vi "GetCoeffsDomains_v1.vi"(0 "R_H coeffs file":path, 1 "Field index":u16, 2 "Fields":string[](array[string]), 5 "R_H domain file":path, 7 "R_C1 coeffs file":path, 9 "R_C1 domain file":path, 11 "R_C2 coeffs file":path, 12 "R_C2 domain file":path) -> (4 "R_H coeffs":dbl[](array[numeric]), 6 "R_H Log Domain":dbl[](array[numeric]), 8 "R_C1 coeffs":dbl[](array[numeric]), 10 "R_C1 Log Domain":dbl[](array[numeric]), 14 "R_C2 Log Domain":dbl[](array[numeric]), 15 "R_C2 coeffs":dbl[](array[numeric]))   [LabVIEW 2020]
uses:
  <vilib>/Utility/file.llb/Read Delimited Spreadsheet (DBL).vi
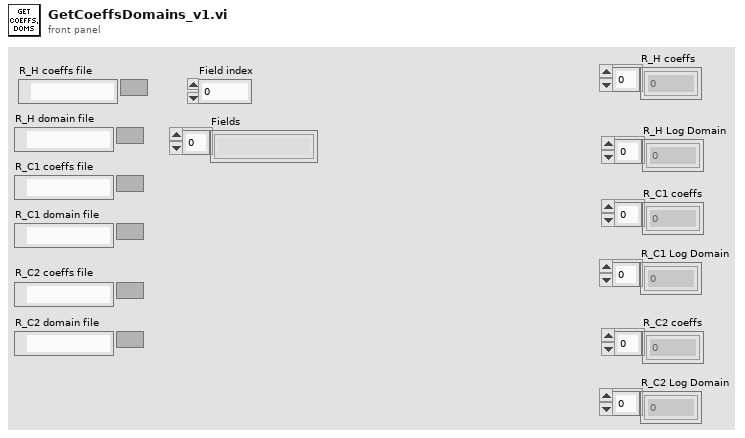
[diagram p1: front panel]
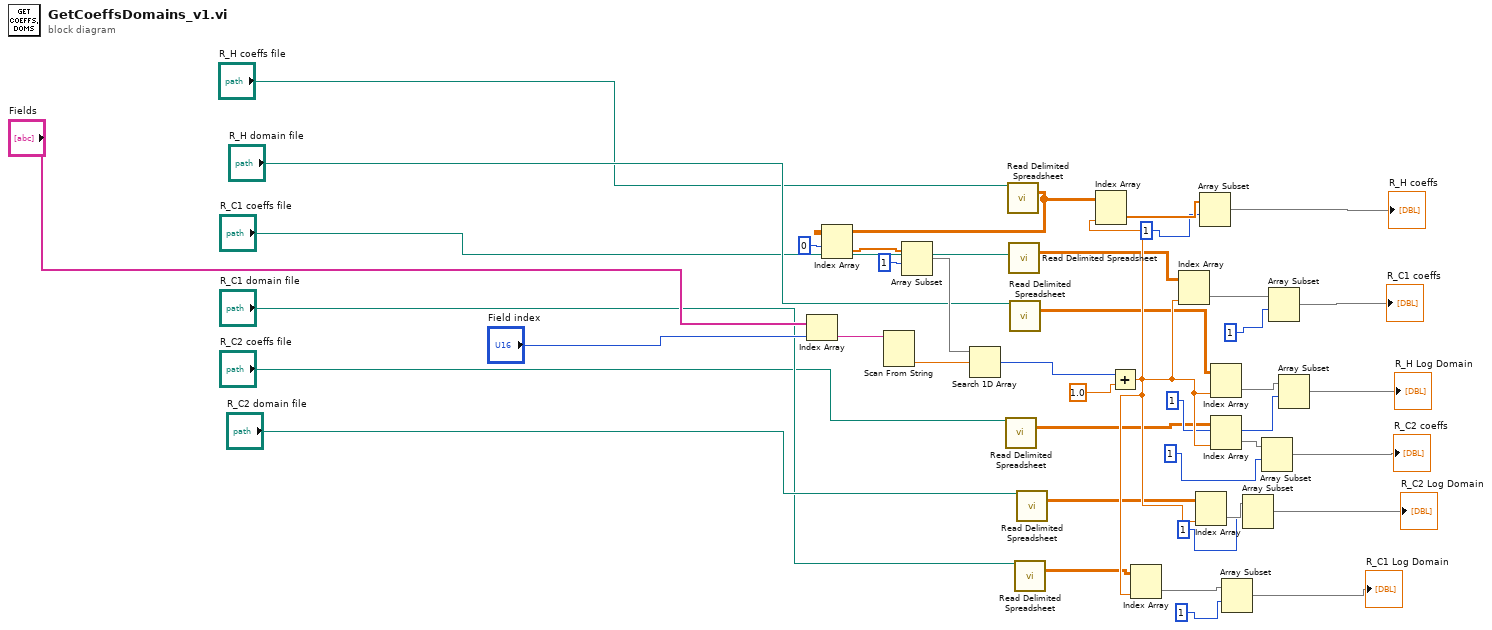
[diagram p0: block diagram]
diagram:
  n1 = Index Array(array="Fields", index="Field index") -> (element=w14:string)
  n2 = Scan From String(input string=w14) -> (output 1=w16:dbl)  [unwired: 4 in, 3 out]
  n3 = call-poly <vilib>:"Read Delimited Spreadsheet.vi"("file path (dialog if empty)"="R_C2 coeffs file") -> ("all rows"=w6:dbl[][])  [unwired: 9 in, 5 out]
  n4 = call-poly <vilib>:"Read Delimited Spreadsheet.vi"("file path (dialog if empty)"="R_H coeffs file") -> ("all rows"=w2:dbl[][])  [unwired: 9 in, 5 out]
  n5 = Index Array(array=w2, index (row)=0) -> (element=w20:dbl[])  [unwired: 1 in]
  n6 = Array Subset(array=w20, index=1) -> (w22:dbl[])  [unwired: 1 in]
  n7 = Search 1D Array(1D array=w22, element=w16) -> (index of element=w24:i32)  [unwired: 1 in]
  n8 = call-poly <vilib>:"Read Delimited Spreadsheet.vi"("file path (dialog if empty)"="R_C1 coeffs file") -> ("all rows"=w4:dbl[][])  [unwired: 9 in, 5 out]
  n9 = call-poly <vilib>:"Read Delimited Spreadsheet.vi"("file path (dialog if empty)"="R_H domain file") -> ("all rows"=w10:dbl[][])  [unwired: 9 in, 5 out]
  n10 = call-poly <vilib>:"Read Delimited Spreadsheet.vi"("file path (dialog if empty)"="R_C1 domain file") -> ("all rows"=w11:dbl[][])  [unwired: 9 in, 5 out]
  n11 = call-poly <vilib>:"Read Delimited Spreadsheet.vi"("file path (dialog if empty)"="R_C2 domain file") -> ("all rows"=w12:dbl[][])  [unwired: 9 in, 5 out]
  n12 = Add(x=w24, y=1.0) -> (x+y=w40:dbl)
  n13 = Index Array(array=w2, index (col)=w40) -> (element=w18:dbl[])  [unwired: 1 in]
  n14 = Index Array(array=w11, index (col)=w40) -> (element=w36:dbl[])  [unwired: 1 in]
  n15 = Index Array(array=w4, index (col)=w40) -> (element=w26:dbl[])  [unwired: 1 in]
  n16 = Index Array(array=w12, index (col)=w40) -> (element=w38:dbl[])  [unwired: 1 in]
  n17 = Array Subset(array=w18, index=1) -> (→"R_H coeffs":dbl[])  [unwired: 1 in]
  n18 = Index Array(array=w10, index (col)=w40) -> (element=w34:dbl[])  [unwired: 1 in]
  n19 = Index Array(array=w6, index (col)=w40) -> (element=w29:dbl[])  [unwired: 1 in]
  n20 = Array Subset(array=w36, index=1) -> (→"R_C1 Log Domain":dbl[])  [unwired: 1 in]
  n21 = Array Subset(array=w38, index=1) -> (→"R_C2 Log Domain":dbl[])  [unwired: 1 in]
  n22 = Array Subset(array=w29, index=1) -> (→"R_C2 coeffs":dbl[])  [unwired: 1 in]
  n23 = Array Subset(array=w26, index=1) -> (→"R_C1 coeffs":dbl[])  [unwired: 1 in]
  n24 = Array Subset(array=w34, index=1) -> (→"R_H Log Domain":dbl[])  [unwired: 1 in]
